vi "Test setExptParam.vi"   [LabVIEW 2019, in "Inst.Transport.lvclass"]
uses:
  Inst.Transport.lvclass
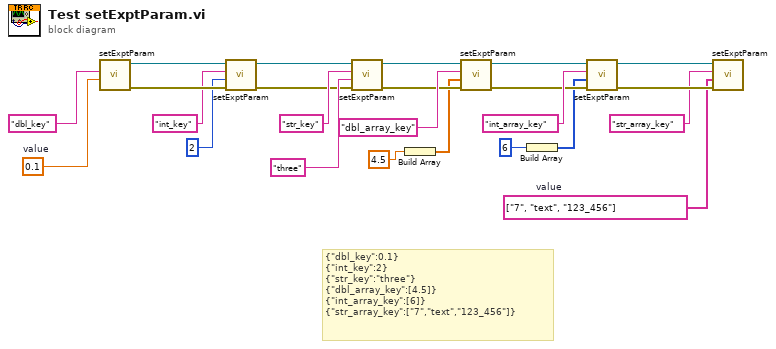
[diagram p0: block diagram]
diagram:
  w1 = string[] ["7", "text", "123_456"]  # value
  w23 = 0.1  # value
  # "{\"dbl_key\":0.1}\n{\"int_key\":2}\n{\"str_key\":\"three\"}\n{\"dbl_array_key\":[4.5]}\n{\"int_array_key\":[6]}\n{\"str_array_key\":[\"7\",\"text\",\"123_456\"]}"
  n1 = call "setExptParam.vi"("value"=w23, "key"="dbl_key") -> ("error out"=w22:errorcluster, "Inst.Transport out"=w21:refnum<class "Inst.Transport.lvclass">)  [unwired: 8 in]
  n2 = call "setExptParam.vi"("error in (no error)"=w22, "value"=2, "key"="int_key", "Inst.Transport in"=w21) -> ("error out"=w16:errorcluster, "Inst.Transport out"=w15:refnum<class "Inst.Transport.lvclass">)  [unwired: 6 in]
  n3 = call "setExptParam.vi"("error in (no error)"=w16, "value"="three", "key"="str_key", "Inst.Transport in"=w15) -> ("error out"=w5:errorcluster, "Inst.Transport out"=w4:refnum<class "Inst.Transport.lvclass">)  [unwired: 6 in]
  n4 = Build Array(4.5) -> (w3:dbl[])
  n5 = call "setExptParam.vi"("error in (no error)"=w5, "value"=w3, "key"="dbl_array_key", "Inst.Transport in"=w4) -> ("error out"=w8:errorcluster, "Inst.Transport out"=w9:refnum<class "Inst.Transport.lvclass">)  [unwired: 6 in]
  n6 = Build Array(6) -> (w2:i32[])
  n7 = call "setExptParam.vi"("error in (no error)"=w8, "value"=w2, "key"="int_array_key", "Inst.Transport in"=w9) -> ("error out"=w13:errorcluster, "Inst.Transport out"=w14:refnum<class "Inst.Transport.lvclass">)  [unwired: 6 in]
  n8 = call "setExptParam.vi"("error in (no error)"=w13, "value"=w1, "key"="str_array_key", "Inst.Transport in"=w14) -> ()  [unwired: 6 in, 2 out]
